vi "PrefDialog.vi"(8 "error in (no error)":errorcluster, 11 "MyPluginsBase in":refnum<class "NHRDCPower.lvclass">) -> (0 "error out":errorcluster, 1 "Save As":bool, 2 "Changed":bool, 3 "MyPluginsBase out":refnum<class "NHRDCPower.lvclass">)   [LabVIEW 2018, in "AcPwrPlugins.lvlib" / "NHRDCPower.lvclass"]
doc: "This VI displays the prior instruments properties and allows a user to change the instrument properties and save these new set properties to the same location on disk or in a new location with a new name called \"Type\"."
uses:
  NHRDCPower.lvclass
  F:/Program Files (x86)/National Instruments/LabVIEW 2018/user.lib/NIST/BaseClasses/BasePlugin_class/BasePlugin.lvclass
  F:/Projects/ICDAS/NistPluggableModules/AcPwr/AcPwrPlugins/AcPwrBaseClass/AcPwrBase.lvclass
  TypeDefs/Device(s)Settings.ctl
  TypeDefs/Modules.ctl
  TypeDefs/Measurements.ctl
  <userlib>/NIST/BaseClasses/BasePlugin_class/BasePlugin.lvclass/BasePlugin.ctl
  AcPwrBaseClass/AcPwrBase.lvclass/AcPwrBase.ctl
  <userlib>/NIST/BaseClasses/BasePlugin_class/Accessors/Read PluginIniFilePath.vi
  AcPwrBaseClass/Accessors/Read BaseConfig.vi
  AcPwrBaseClass/Accessors/Read BaseMeasurements.vi
  <userlib>/NIST/BaseClasses/BasePlugin_class/Accessors/Write PluginIniFilePath.vi
  <vilib>/Utility/error.llb/Error Cluster From Error Code.vi
  <vilib>/ErrorRing/Error Ring.xnode
  <vilib>/Utility/config.llb/NI_LVConfig.lvlib
  AcPwrBaseClass/AcPwrBase.lvclass
  <instrlib>/NHRDCPowerModule/NHRDCPowerModule/NHRDCPowerModule.lvlib
panel:
  in  "uIndex":u32
  in  "btnMacroEdit":bool
  in  "Measurements":T1
  in  "Device(s)Settings":T2 {"Modules"."Regulation Gain (1=100%)" min=0.0 max=1.0; "Modules"."OutputSettings"."Wait on Value" items=["Voltage Greater Than Or Equal To", "Voltage Less Than Or Equal To", "Current Greater Than Or Equal To", "Current Less Than Or Equal To", "Power Greater Than Or Equal To", "Power Less Than Or Equal To"]; "Modules"."operating state (Off)" items=["Off", "Stand By", "Charge", "Discharge", "Battery Emulation"]}
  in  "btnSaveAs":bool
  in  "btnSave":bool
  in  "Measurement RefreshTime (ms)":u32
  in  "btnCancel":bool
  # "*Please ensure that Voltage and Current are selected as the 1st and 2nd Measurement variables, respectively, to correctly plot Voltage vs Current in the visualization VI."
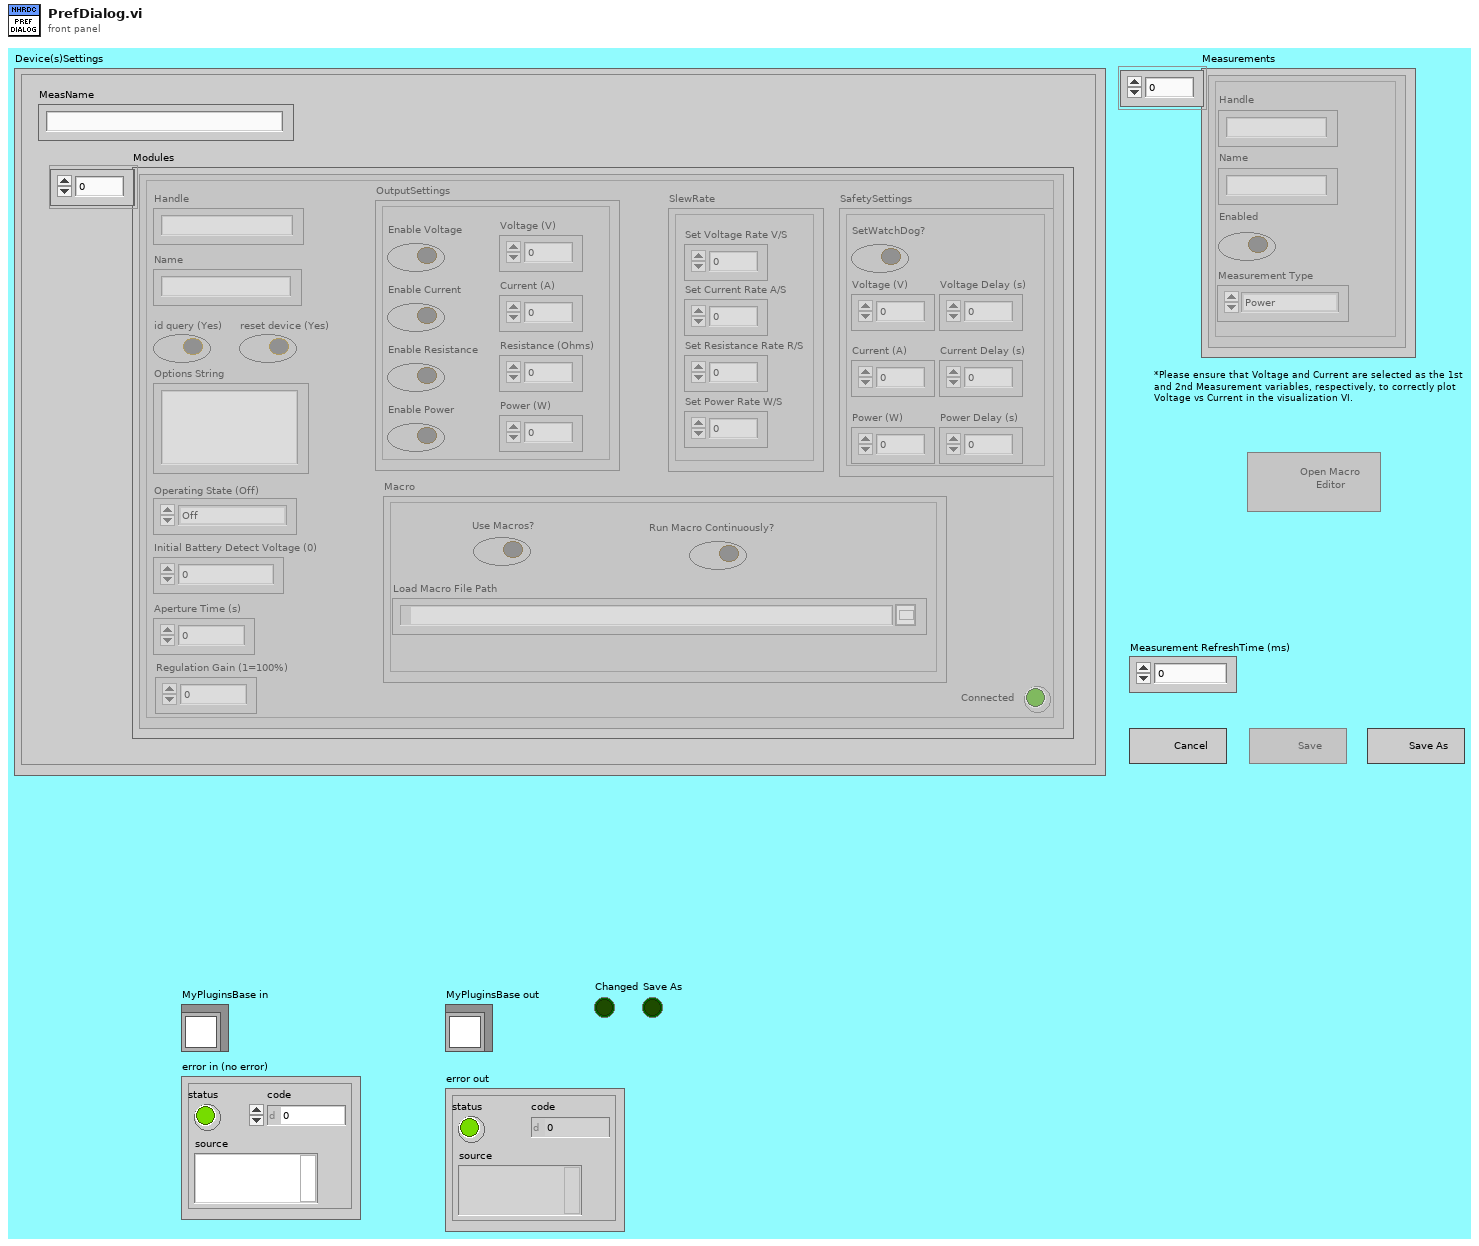
[diagram p1: front panel]
types:
  T1 = typedef "AcPwrPlugins.lvlib/NHRDCPower.lvclass/Measurements.ctl" = cluster{"Handle":string, "Name":string, "Enabled":bool, "Measurement Value":sgl, "Measurement Type":enum16{"Power", "Current", "Voltage"}}[]
  T2 = typedef "AcPwrPlugins.lvlib/NHRDCPower.lvclass/Device(s)Settings.ctl" = cluster{"MeasName":string, "Modules":T3}
  T3 = typedef "AcPwrPlugins.lvlib/NHRDCPower.lvclass/Modules.ctl" = cluster{"Handle":string, "Name":string, "id query (Yes)":bool, "reset device (Yes)":bool, "Connected":bool, "Initial Battery Detect Voltage (0)":dbl, "SafetySettings":cluster{"SetWatchDog?":bool, "Voltage (V)":dbl, "Current (A)":dbl, "Power (W)":dbl, "Voltage Delay (s)":dbl, "Current Delay (s)":dbl, "Power Delay (s)":dbl}, "Options String":string, "Aperture Time (s)":dbl, "operating state (Off)":i32, "OutputSettings":cluster{"Voltage (V)":dbl, "Current (A)":dbl, "Resistance (Ohms)":dbl, "Power (W)":dbl, "Enable Voltage":bool, "Enable Current":bool, "Enable Resistance":bool, "Enable Power":bool, "Macro After Step Delay  (s)":dbl, "Wait Value (V, A, W)":dbl, "Enable Wait":bool, "Wait on Value":i32}, "SlewRate":cluster{"Set Voltage Rate V/S":dbl, "Set Current Rate A/S":dbl, "Set Resistance Rate R/S":dbl, "Set Power Rate W/S":dbl}, "Macro":cluster{"Save Macro?":bool, "Load Macro From File?":bool, "Run Macro Continuously?":bool, "Use Macros?":bool, "Load Macro File Path":path, "Save Macro File Path":string}, "Regulation Gain (1=100%)":dbl, "UpdatingOntheFly":bool}[]
  T4 = enum8{"Enabled", "Disabled", "Disabled and Grayed Out"}
  T5 = enum32{"Invalid", "Standard", "Closed", "Hidden", "Minimized", "Maximized"}
  T6 = enum32{"Invalid", "Default", "Floating", "Floating/Auto-Hide", "Modal"}
  T7 = cluster{"Handle":string, "Name":string, "id query (Yes)":bool, "reset device (Yes)":bool, "Connected":bool, "Initial Battery Detect Voltage (0)":dbl, "SafetySettings":cluster{"SetWatchDog?":bool, "Voltage (V)":dbl, "Current (A)":dbl, "Power (W)":dbl, "Voltage Delay (s)":dbl, "Current Delay (s)":dbl, "Power Delay (s)":dbl}, "Options String":string, "Aperture Time (s)":dbl, "operating state (Off)":i32, "OutputSettings":cluster{"Voltage (V)":dbl, "Current (A)":dbl, "Resistance (Ohms)":dbl, "Power (W)":dbl, "Enable Voltage":bool, "Enable Current":bool, "Enable Resistance":bool, "Enable Power":bool, "Macro After Step Delay  (s)":dbl, "Wait Value (V, A, W)":dbl, "Enable Wait":bool, "Wait on Value":i32}, "SlewRate":cluster{"Set Voltage Rate V/S":dbl, "Set Current Rate A/S":dbl, "Set Resistance Rate R/S":dbl, "Set Power Rate W/S":dbl}, "Macro":cluster{"Save Macro?":bool, "Load Macro From File?":bool, "Run Macro Continuously?":bool, "Use Macros?":bool, "Load Macro File Path":path, "Save Macro File Path":string}, "Regulation Gain (1=100%)":dbl, "UpdatingOntheFly":bool}
  T8 = typedef "AcPwrPlugins.lvlib/AcPwrBase.lvclass/BaseConfig.ctl" = cluster{"Frequency":dbl, "FrequencyRange":dbl[], "Phases":T9[], "Name":string, "PluginConfigVariant":variant, "PluginMeasVariant":variant}
  T9 = typedef "AcPwrPlugins.lvlib/AcPwrBase.lvclass/Phase.ctl" = cluster{"Name":string, "Enabled":bool, "VoltageLevel":dbl, "Handle":string, "VoltageRange":dbl[], "Connected":bool, "CurrentLimit":dbl, "Waveform":string}
  T10 = typedef "AcPwrPlugins.lvlib/AcPwrBase.lvclass/BaseMeasurements.ctl" = cluster{"Handle":string, "Name":string, "Enabled":bool, "Measurement Value":dbl, "btnMeasFetch":bool, "Chroma Hold Peak Current Measurement":bool, "Chroma Measurement Type":T11, "Chroma Protection Status String":string, "NHRDC Fetch Method":i32, "NHRDC Fetch Time (s)":sgl, "NHRDC Measurement Type":i32, "NHRGridSim Measurement Type ":enum16{"Average Current", "Max Current", "Min Current", "Average Voltage", "Max Voltage", "Min Voltage", "Average True Power", "Max True Power", "Min True Power", "Average Apparent Power", "Max Apparent Power", "Min Apparent Power", "Power Factor", "Crest Factor"}, "NHRGridSim Phase ":i32, "PPS Measurement Type ":enum16{"Voltage RMS L-N", "Voltage RMS L-L", "Frequency", "Current RMS", "Current Peak", "Crest Factor", "Power Factor", "Power VA", "Real Power"}, "PPS Channel Name":enum16{"A", "B", "C"}}[]
  T11 = typedef "AcPwrPlugins.lvlib/ChromaAcLoad.lvclass/MeasurementType.ctl" = enum16{"Voltage (Vrms or V)", "Current (Arms or A)", "Power (W)", "Peak Voltage (V)", "Peak Current (A)", "Peak Power (W)", "Frequency (Hz)", "Resistance (Ohms)", "Voltage Overshoot (V)", "Positive Peak Current (A)", "Voltage Undershoot (V)", "Negative Peak Current (A)", "Apparent Power (VA)", "Reacitive Power (VAR)", "Voltage THD", "Power Factor", "Current's Crest Factor"}
  T12 = typedef "NI_LVConfig.lvlib/Config Data RefNum.ctl" = refnum<k1>
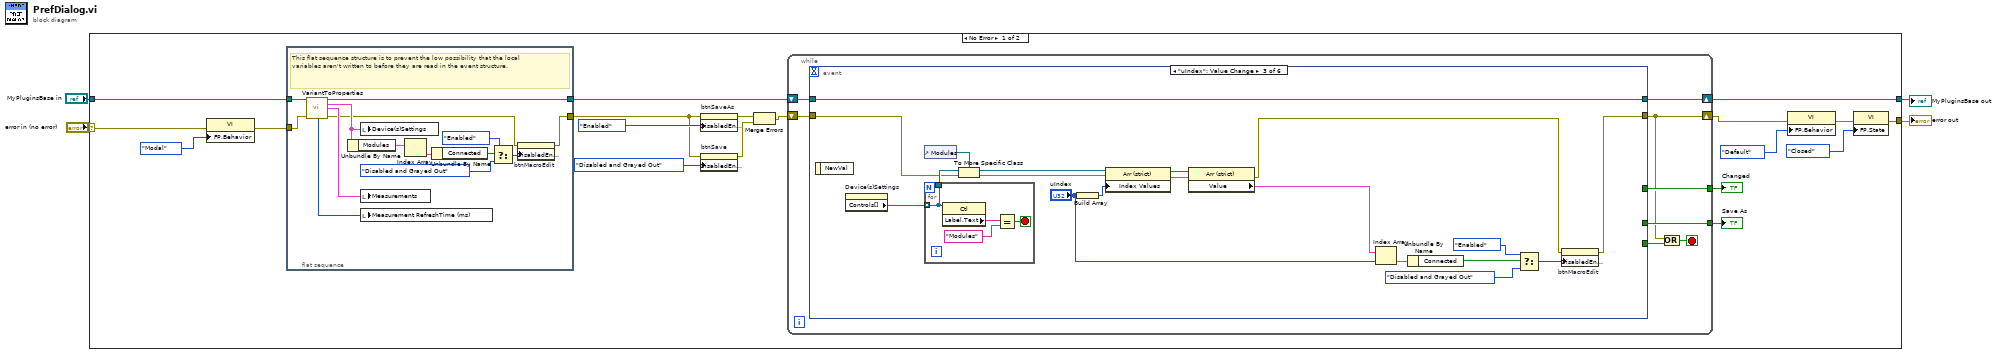
[diagram p0: block diagram]
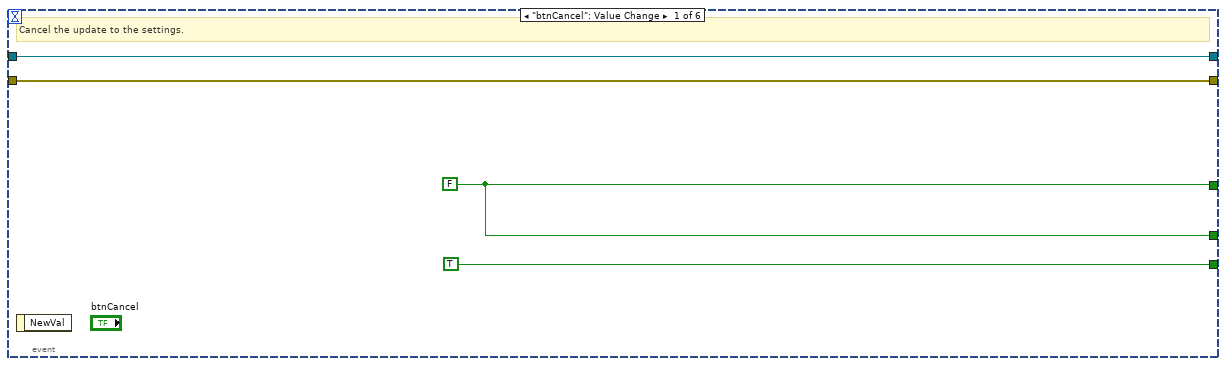
[diagram p2: hidden frame]
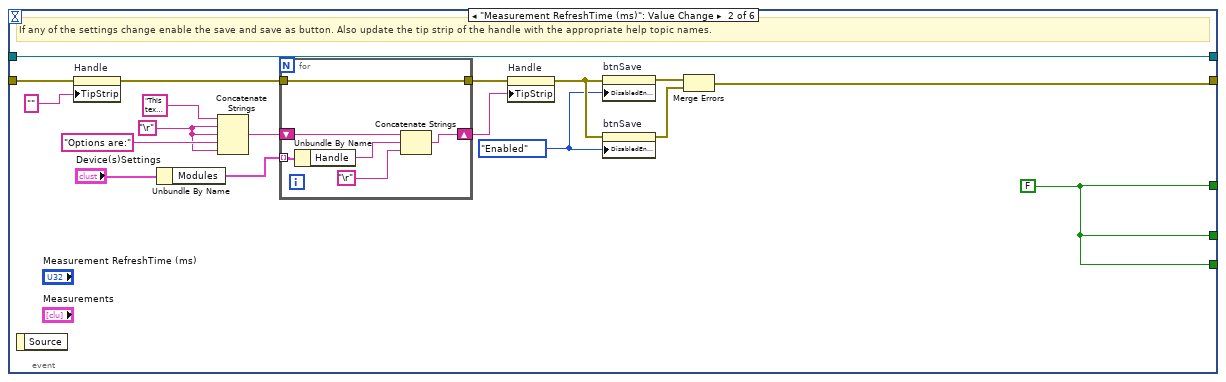
[diagram p3: hidden frame]
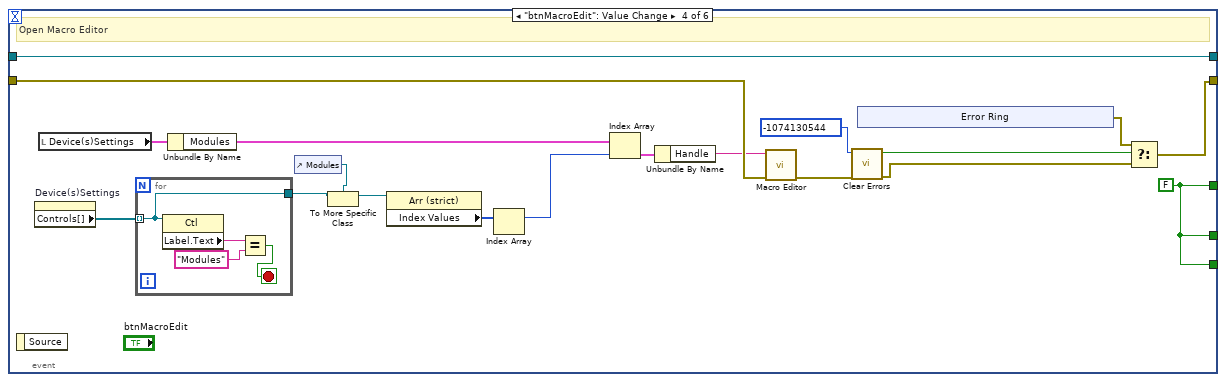
[diagram p4: hidden frame]
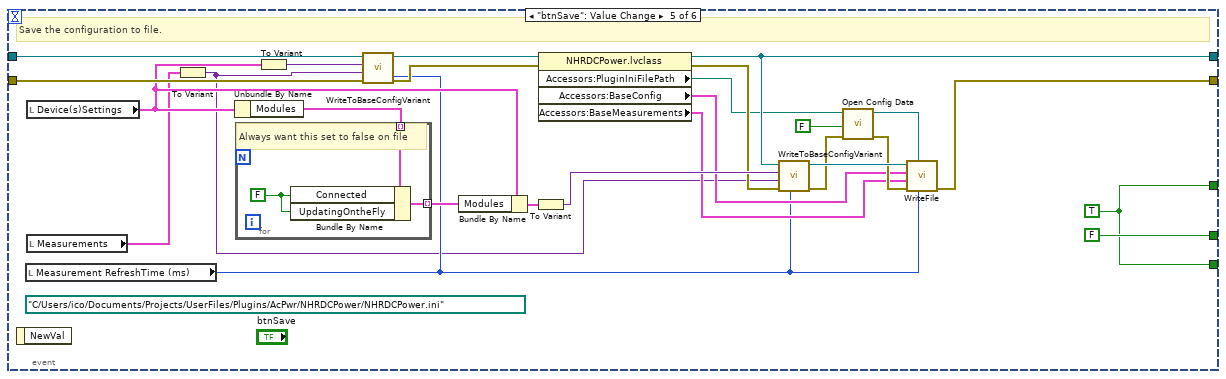
[diagram p5: hidden frame]
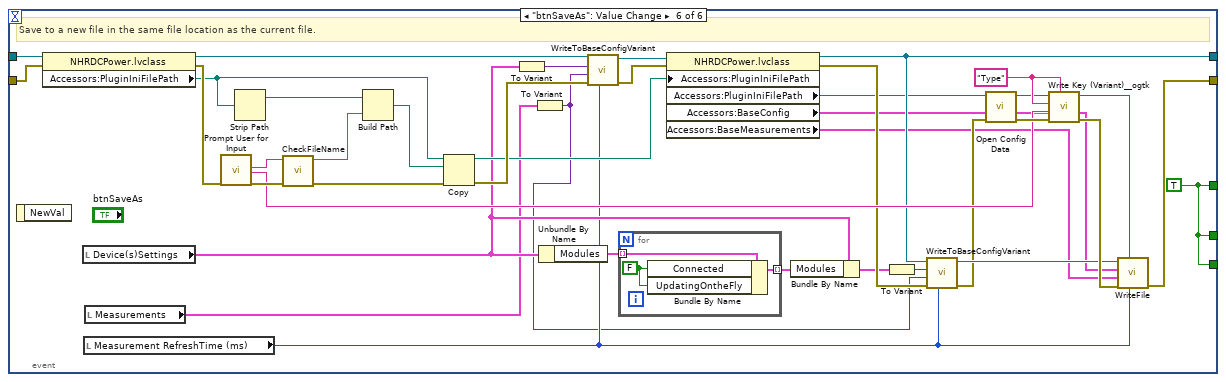
[diagram p6: hidden frame]
diagram:
  n1 = case shown="No Error" "error in (no error)" {
    selector: "error in (no error)" -> [w6 w197]
    tunnel: "MyPluginsBase in" -> [w19 w196]
    tunnel: [w17 w196] -> w2
    tunnel: [w16 w197] -> w1
    frame No Error {
      n2 = property class="VI"(error in=w6, "FP.Behavior"=T6."Modal" ("Front Panel Window:Behavior")) -> (error out=w5:errorcluster)  [unwired: 1 in, 1 out]
      n3 = flat-sequence {
        tunnel: w19 -> [w37]
        tunnel: [w35] -> w18
        tunnel: [w24] -> w8
        tunnel: w5 -> [w36]
        frame #0 {
          # "This flat sequence structure is to prevent the low possibility that the local variables aren't written to before they are read in the event structure."
          n4 = call "VariantToProperties.vi"("NHRDCPower in"=w37, "error in (no error)"=w36) -> ("NHRDCPower out"=w35:refnum<class "NHRDCPower.lvclass">, "NHRDC"=w32:T2, "Meas"=w34:T1, "Measurement Refresh Time (ms)"=w33:u32, "error out"=w25:errorcluster)  [unwired: 7 in, 2 out]
          n5 = Unbundle By Name(w32) -> ("Modules"=w31:T3)
          n6 = local write "Device(s)Settings"(w32) -> ()
          n7 = local write "Measurements"(w34) -> ()
          n8 = local write "Measurement RefreshTime (ms)"(w33) -> ()
          n9 = Index Array(array=w31) -> (element=w30:T7)  [unwired: 1 in]
          n10 = Unbundle By Name(w30) -> ("Connected"=w29:bool)
          n11 = Select(t=T4."Enabled" ("Disabled"), s=w29, f=T4."Disabled and Grayed Out" ("Disabled")) -> (s? t:f=w26:T4)
          n12 = property on="btnMacroEdit" class="Bool"(error in=w25, "DisabledEnum"=w26) -> (error out=w24:errorcluster)  [unwired: 1 in, 1 out]
        }
      }
      n13 = property on="btnSaveAs" class="Bool"(error in=w8, "DisabledEnum"=T4."Enabled" ("Disabled")) -> (error out=w11:errorcluster)  [unwired: 1 in, 1 out]
      n14 = property on="btnSave" class="Bool"(error in=w8, "DisabledEnum"=T4."Disabled and Grayed Out" ("Disabled")) -> (error out=w10:errorcluster)  [unwired: 1 in, 1 out]
      n15 = Merge Errors(w11, w10) -> (w14:errorcluster)
      n16 = while {
        shift-right: [w42] -> w17
        shift-left: w18 -> [w43]
        tunnel: [w45] -> w13
        tunnel: [w40] -> w12
        shift-right: [w38] -> w15
        shift-left: w14 -> [w41]
        stop <- w39 stop-if-true
        n17 = event shown="[2] \"uIndex\": Value Change" {
          selector: _ -> [_ _ _ _ _ _]
          dyn-events: _ -> [_ _ _ _ _ _]
          timeout: _ -> [_ _ _ _ _ _]
          tunnel: [w46 w66 _ w101 w149 w190] -> w45
          tunnel: [TRUE w66 _ w101 w149 w190] -> w44
          tunnel: w43 -> [w48 w67 w88 w115 w147 w183]
          tunnel: [w48 w67 w88 w115 w133 w172] -> w42
          tunnel: [w47 w65 w86 w97 w148 w176] -> w38
          tunnel: w41 -> [w47 w52 w75 w111 w146 w182]
          tunnel: [w46 w66 _ w101 FALSE w190] -> w40
          event "btnCancel": Value Change {
            w46 = FALSE
            # "Cancel the update to the settings."
            n18 = event-data() -> ()  [unwired: 1 in, 1 out]
          }
          event "Measurement RefreshTime (ms)": Value Change {
            w53 = T4."Enabled" ("Disabled")
            w62 = "\r"
            w66 = FALSE
            # "If any of the settings change enable the save and save as button. Also update the tip strip of the handle with the appropriate help topic names."
            n19 = event-data() -> ()  [unwired: 1 in, 1 out]
            n20 = property on="Handle" class="Str"(error in=w52, "TipStrip"="" ("Tip Strip")) -> (error out=w57:errorcluster)  [unwired: 1 in, 1 out]
            n21 = Unbundle By Name("Device(s)Settings") -> ("Modules"=w50:T3)
            n22 = Concatenate Strings("This text in this handle of the instrument and entered in the  \nhandle control in the Phases array EXACTLY, lest the attempt \nto interact with the instrument will fail.", w62, w62, "Options are:" ("Handle"), w62) -> (w61:string)
            n23 = for {
              shift-right: [w73] -> w60
              shift-left: w61 -> [w72]
              tunnel: w57 -> [w70]
              tunnel: [w70] -> w56
              tunnel: w50 -> [w69] mode=indexing
              n24 = Unbundle By Name(w69) -> ("Handle"=w68:string)
              n25 = Concatenate Strings(w72, w68, "\r") -> (w73:string)
            }
            n26 = property on="Handle" class="Str"(error in=w56, "TipStrip"=w60) -> (error out=w58:errorcluster)  [unwired: 1 in, 1 out]
            n27 = property on="btnSave" class="Bool"(error in=w58, "DisabledEnum"=w53) -> (error out=w55:errorcluster)  [unwired: 1 in, 1 out]
            n28 = property on="btnSave" class="Bool"(error in=w58, "DisabledEnum"=w53) -> (error out=w54:errorcluster)  [unwired: 1 in, 1 out]
            n29 = Merge Errors(w55, w54) -> (w65:errorcluster)
          }
          event "uIndex": Value Change {
            n30 = event-data() -> ()  [unwired: 1 in, 1 out]
            n31 = property on="Device(s)Settings" class="Clust (strict)"() -> ("Controls[]"=w82:refnum<vi>[])  [unwired: 2 in, 2 out]
            n32 = control-ref of="Modules"() -> (w84:refnum<vi>)
            n33 = for {
              tunnel: w82 -> [w93] mode=indexing
              tunnel: [w93] -> w83
              stop <- w94 stop-if-true
              n34 = property class="Ctl"(reference=w93) -> ("Label.Text"=w96:string)  [unwired: 1 in, 2 out]
              n35 = Equal?(x=w96, y="Modules") -> (x = y?=w94:bool)
            }
            n36 = To More Specific Class(target class=w84, reference=w83, error in=w75) -> (specific class reference=w85:refnum<vi>, error out=w74:errorcluster)
            n37 = Build Array("uIndex") -> (w81:u32[])
            n38 = property class="Arr (strict)"(reference=w85, error in=w74, "Index Values"=w81) -> (reference out=w79:refnum<vi>, error out=w78:errorcluster)
            n39 = property class="Arr (strict)"(reference=w79, error in=w78) -> (error out=w76:errorcluster, "Value"=w77:T3)  [unwired: 1 out]
            n40 = Index Array(array=w77, index="uIndex") -> (element=w92:T7)
            n41 = Unbundle By Name(w92) -> ("Connected"=w91:bool)
            n42 = Select(t=T4."Enabled" ("Disabled"), s=w91, f=T4."Disabled and Grayed Out" ("Disabled")) -> (s? t:f=w87:T4)
            n43 = property on="btnMacroEdit" class="Bool"(error in=w76, "DisabledEnum"=w87) -> (error out=w86:errorcluster)  [unwired: 1 in, 1 out]
          }
          event "btnMacroEdit": Value Change {
            w101 = FALSE
            # "Open Macro Editor"
            n44 = event-data() -> ()  [unwired: 1 in, 1 out]
            n45 = property on="Device(s)Settings" class="Clust (strict)"() -> ("Controls[]"=w114:refnum<vi>[])  [unwired: 2 in, 2 out]
            n46 = local read "Device(s)Settings"() -> (w113:T2)
            n47 = for {
              tunnel: w114 -> [w121] mode=indexing
              tunnel: [w121] -> w110
              stop <- w122 stop-if-true
              n48 = property class="Ctl"(reference=w121) -> ("Label.Text"=w124:string)  [unwired: 1 in, 2 out]
              n49 = Equal?(x=w124, y="Modules") -> (x = y?=w122:bool)
            }
            n50 = Unbundle By Name(w113) -> ("Modules"=w112:T3)
            n51 = control-ref of="Modules"() -> (w109:refnum<vi>)
            n52 = To More Specific Class(target class=w109, reference=w110) -> (specific class reference=w108:refnum<vi>)  [unwired: 1 in, 1 out]
            n53 = property class="Arr (strict)"(reference=w108) -> ("Index Values"=w107:u32[])  [unwired: 1 in, 2 out]
            n54 = Index Array(array=w107) -> (element=w106:u32)  [unwired: 1 in]
            n55 = Index Array(array=w112, index=w106) -> (element=w105:T7)
            n56 = Unbundle By Name(w105) -> ("Handle"=w104:string)
            n57 = call <instrlib>:"Macro Editor.vi"("error in (no error)"=w111, "instrument handle"=w104) -> ("error out"=w103:errorcluster)  [unwired: 7 in, 2 out]
            n58 = call <vilib>:"Clear Errors.vi"("error in (no error)"=w103, "specific error code to clear (0: all)"=-1074130544 ("error code (no error:0)")) -> ("error out"=w98:errorcluster, "specific error cleared?"=w100:bool)  [unwired: 4 in]
            n59 = xnode "Error Ring"() -> ("error out"=w99:errorcluster)
            n60 = Select(t=w99, s=w100, f=w98) -> (s? t:f=w97:errorcluster)
          }
          event "btnSave": Value Change {
            (unwired) path "C:/Users/ico/Documents/Projects/UserFiles/Plugins/AcPwr/NHRDCPower/NHRDCPower.ini" ("configuration file path")
            w149 = TRUE ("StartMeas")
            # "Save the configuration to file."
            n61 = event-data() -> ()  [unwired: 1 in, 1 out]
            n62 = local read "Measurement RefreshTime (ms)"() -> (w127:u32)
            n63 = local read "Device(s)Settings"() -> (w136:T2)
            n64 = local read "Measurements"() -> (w126:T1)
            n65 = To Variant(anything=w126) -> (Variant=w125:variant)
            n66 = Unbundle By Name(w136) -> ("Modules"=w141:T3)
            n67 = for {
              tunnel: [w153] -> w137 mode=indexing
              tunnel: w141 -> [w152] mode=indexing
              w151 = FALSE ("Connected")
              # "Always want this set to false on file"
              n68 = Bundle By Name(cluster=w152, "Connected"=w151, "UpdatingOntheFly"=w151) -> (w153:T7)
            }
            n69 = To Variant(anything=w136) -> (Variant=w145:variant)
            n70 = call-dynamic "WriteToBaseConfigVariant.vi"("Measurement Refresh Time (ms)"=w127, "error in (no error)"=w146, "Meas"=w125, "Config"=w145, "NHRDCPower in"=w147) -> ("error out"=w134:errorcluster, "NHRDCPower out"=w143:refnum<class "NHRDCPower.lvclass">)  [unwired: 5 in]
            n71 = Bundle By Name(cluster=w136, "Modules"=w137) -> (w135:T2)
            n72 = To Variant(anything=w135) -> (Variant=w144:variant)
            n73 = property class="NHRDCPower.lvclass"(reference=w143, error in=w134) -> (reference out=w133:refnum<class "NHRDCPower.lvclass">, error out=w132:errorcluster, "Accessors:PluginIniFilePath"=w130:path, "Accessors:BaseConfig"=w129:T8, "Accessors:BaseMeasurements"=w128:T10)
            n74 = call-dynamic "WriteToBaseConfigVariant.vi"("Measurement Refresh Time (ms)"=w127, "error in (no error)"=w132, "Meas"=w125, "Config"=w144, "NHRDCPower in"=w133) -> ("error out"=w131:errorcluster, "NHRDCPower out"=w142:refnum<class "NHRDCPower.lvclass">)  [unwired: 5 in]
            n75 = call <vilib>:"Open Config Data.vi"("error in (no error)"=w131, "create file if necessary (T)"=FALSE, "configuration file path"=w130) -> ("error out"=w139:errorcluster, "refnum"=w138:T12)  [unwired: 6 in, 1 out]
            n76 = call-dynamic "WriteFile.vi"("RefreshTime"=w127, "Refnum in"=w138, "error in (no error)"=w139, "BaseMeasurements"=w128, "BaseConfiguration"=w129, "NHRDCPower in"=w142) -> ("error out"=w148:errorcluster)  [unwired: 4 in, 1 out]
          }
          event "btnSaveAs": Value Change {
            w186 = "Type" ("section (optional)")
            w190 = TRUE
            # "Save to a new file in the same file location as the current file."
            n77 = event-data() -> ()  [unwired: 1 in, 1 out]
            n78 = property class="NHRDCPower.lvclass"(reference=w183, error in=w182) -> (reference out=w164:refnum<class "NHRDCPower.lvclass">, error out=w181:errorcluster, "Accessors:PluginIniFilePath"=w179:path)
            n79 = local read "Device(s)Settings"() -> (w160:T2)
            n80 = local read "Measurement RefreshTime (ms)"() -> (w157:u32)
            n81 = local read "Measurements"() -> (w155:T1)
            n82 = call "Prompt User for Input"("error in (no error)"=w181) -> ("File Name"=w180:string, "PluginType"=w178:string, "error out"=w187:errorcluster)  [unwired: 15 in, 1 out]
            n83 = Strip Path(path=w179) -> (stripped path=w192:path)  [unwired: 1 out]
            n84 = call "CheckFileName.vi"("Error In"=w187, "File Name in"=w180) -> ("Error Out"=w188:errorcluster, "File Name out"=w189:string)  [unwired: 8 in]
            n85 = Build Path(base path=w192, name or relative path=w189) -> (appended path=w191:path)
            n86 = Copy(8:w188, 10:w191, 11:w179) -> (0:w162:errorcluster, 3:w161:path)  [unwired: 2 in, 1 out]
            n87 = To Variant(anything=w160) -> (Variant=w166:variant)
            n88 = To Variant(anything=w155) -> (Variant=w154:variant)
            n89 = Unbundle By Name(w160) -> ("Modules"=w169:T3)
            n90 = call-dynamic "WriteToBaseConfigVariant.vi"("Measurement Refresh Time (ms)"=w157, "error in (no error)"=w162, "Meas"=w154, "Config"=w166, "NHRDCPower in"=w164) -> ("error out"=w163:errorcluster, "NHRDCPower out"=w165:refnum<class "NHRDCPower.lvclass">)  [unwired: 5 in]
            n91 = for {
              tunnel: w169 -> [w195] mode=indexing
              tunnel: [w194] -> w168 mode=indexing
              w193 = FALSE ("Connected")
              n92 = Bundle By Name(cluster=w195, "Connected"=w193, "UpdatingOntheFly"=w193) -> (w194:T7)
            }
            n93 = property class="NHRDCPower.lvclass"(reference=w165, error in=w163, "Accessors:PluginIniFilePath"=w161) -> (reference out=w172:refnum<class "NHRDCPower.lvclass">, error out=w171:errorcluster, "Accessors:PluginIniFilePath"=w159:path, "Accessors:BaseConfig"=w158:T8, "Accessors:BaseMeasurements"=w156:T10)
            n94 = Bundle By Name(cluster=w160, "Modules"=w168) -> (w167:T2)
            n95 = To Variant(anything=w167) -> (Variant=w174:variant)
            n96 = call-dynamic "WriteToBaseConfigVariant.vi"("Measurement Refresh Time (ms)"=w157, "error in (no error)"=w171, "Meas"=w154, "Config"=w174, "NHRDCPower in"=w172) -> ("error out"=w170:errorcluster, "NHRDCPower out"=w173:refnum<class "NHRDCPower.lvclass">)  [unwired: 5 in]
            n97 = call <vilib>:"Open Config Data.vi"("error in (no error)"=w170, "configuration file path"=w159) -> ("error out"=w184:errorcluster, "refnum"=w185:T12)  [unwired: 7 in, 1 out]
            n98 = call <userlib>:"Write Key (Variant)__ogtk.vi"("section"=w186, "error in (no error)"=w184, "key-value"=w178, "key (optional)"=w186, "refnum"=w185) -> ("error out"=w177:errorcluster, "refnum out"=w175:T12)  [unwired: 5 in]
            n99 = call-dynamic "WriteFile.vi"("RefreshTime"=w157, "Refnum in"=w175, "error in (no error)"=w177, "BaseMeasurements"=w156, "BaseConfiguration"=w158, "NHRDCPower in"=w173) -> ("error out"=w176:errorcluster)  [unwired: 4 in, 1 out]
          }
        }
        n100 = Or(x=w38, y=w44) -> (x .or. y?=w39:bool)
      }
      "Save As" <- w12
      "Changed" <- w13
      n101 = property class="VI"(error in=w15, "FP.Behavior"=T6."Default" ("Front Panel Window:Behavior")) -> (error out=w22:errorcluster)  [unwired: 1 in, 1 out]
      n102 = property class="VI"(error in=w22, "FP.State"=T5."Closed" ("Front Panel Window:State")) -> (error out=w16:errorcluster)  [unwired: 1 in, 1 out]
    }
    frame Error {
    }
  }
  "error out" <- w1
  "MyPluginsBase out" <- w2
